vi "Read daemon error.vi"(8 "error in (no error)":errorcluster, 11 "Network Slave in":refnum<class "Network Slave.lvclass">) -> (0 "error out":errorcluster, 2 "daemon error":errorcluster, 3 "Network Slave out":refnum<class "Network Slave.lvclass">)   [LabVIEW 2013, in "Modbus Library - Advance.lvlib" / "Network Slave.lvclass"]
uses:
  Network Slave.lvclass
  Network Slave.lvclass/Network Slave.ctl
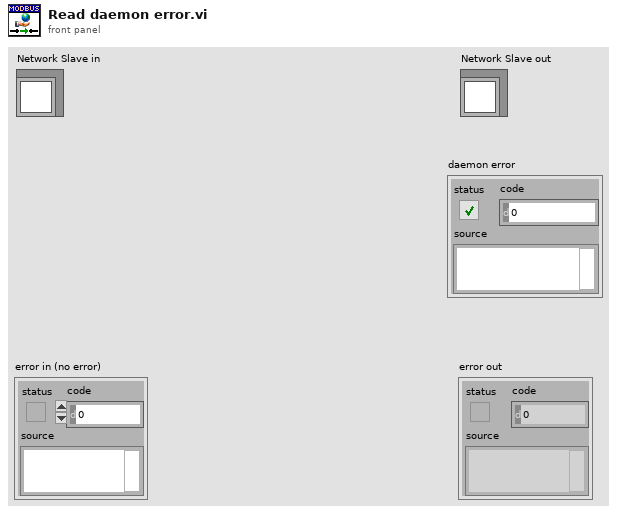
[diagram p1: front panel]
types:
  T1 = typedef "Network Slave.lvclass/daemon status cluster.ctl" = cluster{"error":errorcluster, "status":T2}
  T2 = typedef "Network Slave.lvclass/daemon status.ctl" = enum16{"Not Started", "Running", "Error", "Stopped"}
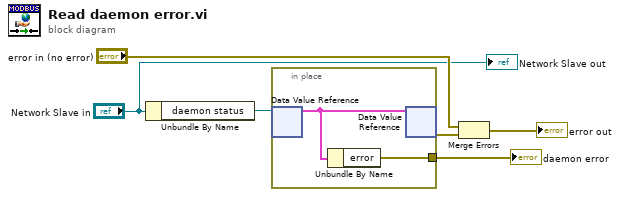
[diagram p0: block diagram]
diagram:
  n1 = Unbundle By Name("Network Slave in") -> ("daemon status"=w5:refnum<data-value>)
  n2 = in-place {
    in-place-border: [w7] -> w1
    n3 = in-place-dvr #1(w5) -> (w8:T1)  [unwired: 1 out]
    n4 = Unbundle By Name(w8) -> ("error"=w7:errorcluster)
    n5 = in-place-dvr #1(w8) -> (w6:errorcluster)  [unwired: 1 out]
  }
  "daemon error" <- w1
  n6 = Merge Errors("error in (no error)", w6) -> (→"error out":errorcluster)
  "Network Slave out" <- "Network Slave in"
